vi "Target.vi"   [LabVIEW 2025]
uses:
  <vilib>/eio/utilities/niEioResolveVilibRelativePath.vi
  <vilib>/rvi/interface/RandomDataEmulation/niFpgaRandomDataHandleErrors.vi
  <vilib>/rvi/Memory/Memory_Emulation/nirvimemoryFastEmulation.vi
  <vilib>/rvi/Memory/Memory_Emulation/nirvimemoryEmulation.vi
  <vilib>/rvi/Emulation/niFpgaEmulationIsFPGAContextNoSignature.vi
  <vilib>/rvi/DataTransferAndStorage/Container/Common/niFpgaContainerGetUniqueNameForEmu.vi
  <vilib>/rvi/Emulation/niFpgaProcessEmulError.vi
  <vilib>/rvi/Emulation/niFpgaSctlEmulationGetInTimedLoop.vi
  <vilib>/rvi/errors/nirviReportUnexpectedCaseInternalError (U32).vi
  <vilib>/ARTS-Lab/Array-based Linear Algebra/vector_matrix_multiply_VIs/vector_matrix_multiply_SGL.vi
  <vilib>/ARTS-Lab/Array-based Linear Algebra/matrix_matrix_VIs/matrix_matrix_multiply_SGL.vi
  <vilib>/rvi/DataTransferAndStorage/Container/XNode/niFpgaContainer.xnode
  <vilib>/rvi/interface/RandomDataEmulation/nirviRandomDataFpgaReadWriteTemplate.vi
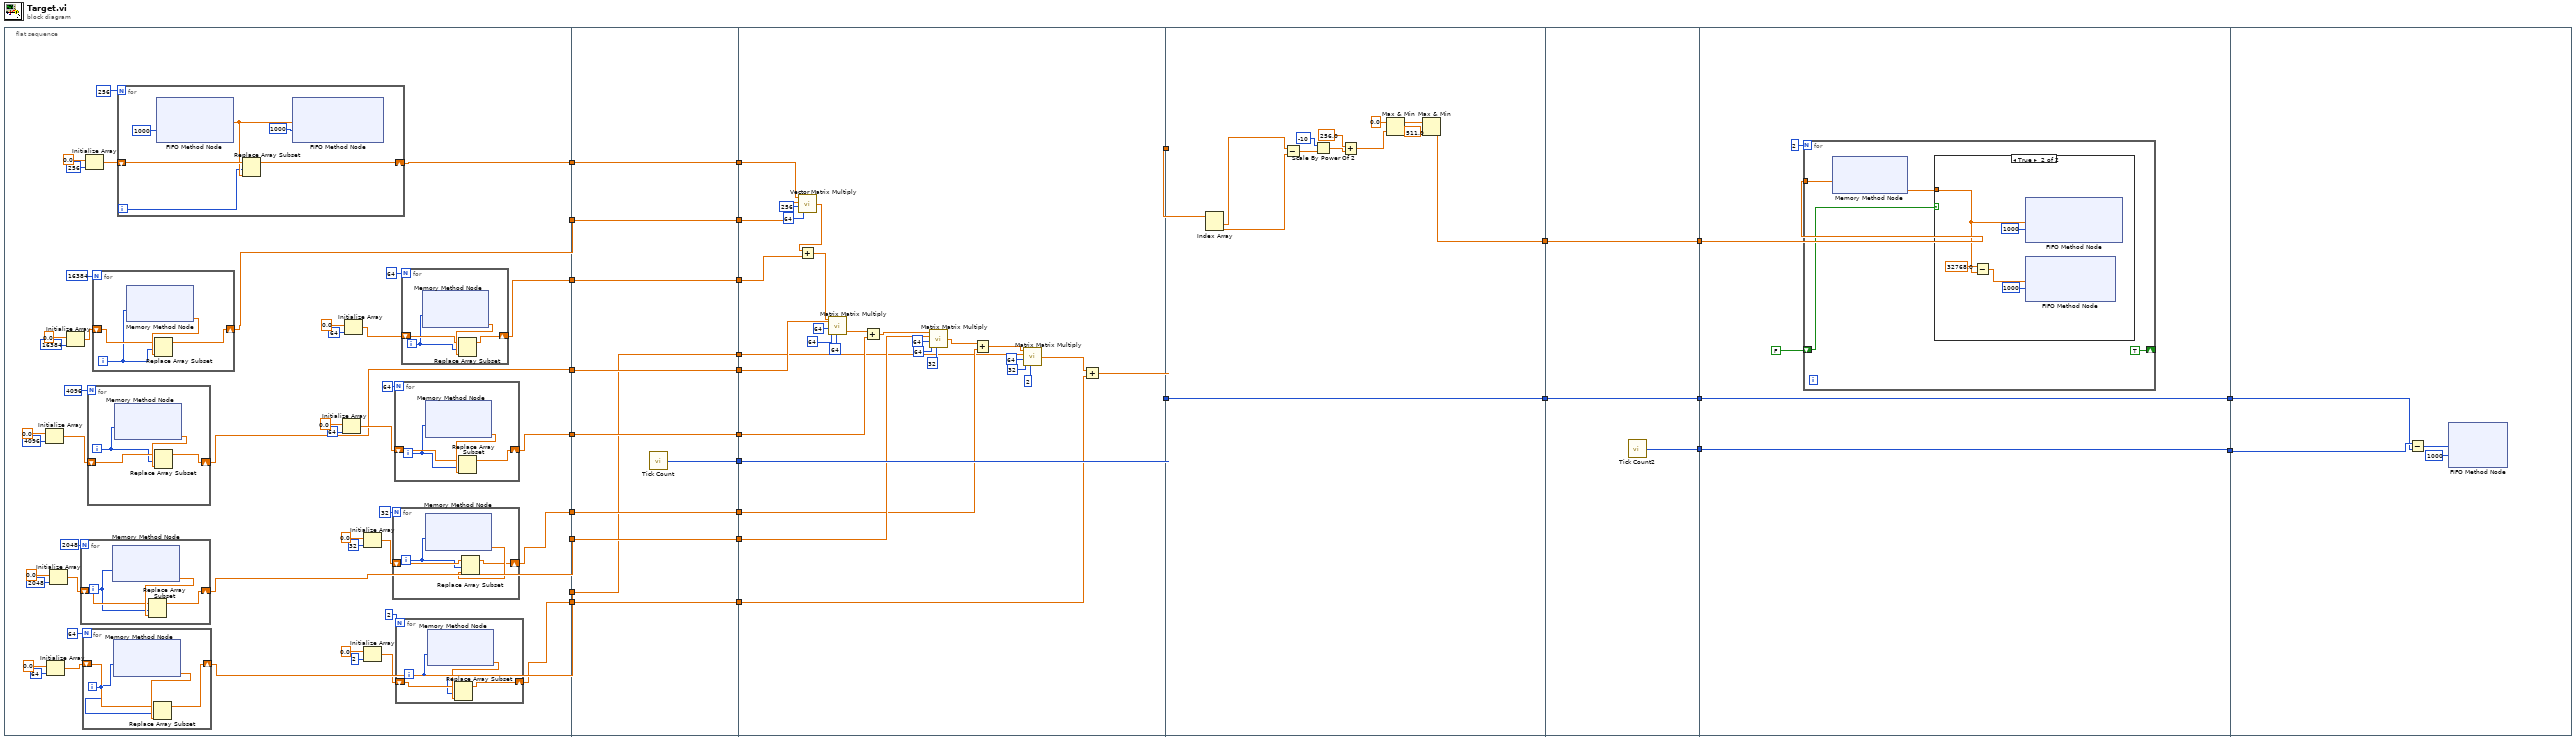
[diagram p0: block diagram]
diagram:
  n1 = flat-sequence {
    tunnel: [w72] -> w19
    tunnel: [w58] -> w17
    tunnel: [w41] -> w15
    tunnel: [w36] -> w13
    tunnel: [w40] -> w11
    tunnel: [w39] -> w8
    tunnel: [w33] -> w6
    tunnel: [w35] -> w4
    tunnel: [w34] -> w1
    tunnel: w19 -> [w121]
    tunnel: [w121] -> w18
    tunnel: w17 -> [w120]
    tunnel: [w120] -> w16
    tunnel: w15 -> [w119]
    tunnel: [w119] -> w14
    tunnel: w13 -> [w118]
    tunnel: [w118] -> w12
    tunnel: w11 -> [w117]
    tunnel: [w117] -> w10
    tunnel: [w116] -> w9
    tunnel: w8 -> [w115]
    tunnel: [w115] -> w7
    tunnel: w6 -> [w114]
    tunnel: [w114] -> w5
    tunnel: w4 -> [w113]
    tunnel: [w113] -> w3
    tunnel: [w112] -> w2
    tunnel: w1 -> [w112]
    tunnel: [w122] -> w28
    tunnel: [w150] -> w27
    tunnel: w9 -> [w150]
    tunnel: w10 -> [w139]
    tunnel: w12 -> [w147]
    tunnel: w14 -> [w141]
    tunnel: w16 -> [w148]
    tunnel: w18 -> [w149]
    tunnel: w7 -> [w136]
    tunnel: w5 -> [w130]
    tunnel: w3 -> [w126]
    tunnel: w2 -> [w125]
    tunnel: w28 -> [w153]
    tunnel: [w152] -> w26
    tunnel: w27 -> [w151]
    tunnel: [w151] -> w25
    tunnel: w26 -> [w166]
    tunnel: [w166] -> w24
    tunnel: w25 -> [w165]
    tunnel: [w165] -> w23
    tunnel: [w164] -> w22
    tunnel: w24 -> [w170]
    tunnel: [w167] -> w21
    tunnel: w23 -> [w168]
    tunnel: [w168] -> w20
    tunnel: w22 -> [w167]
    tunnel: w21 -> [w184]
    tunnel: w20 -> [w183]
    frame #0 {
      n2 = Initialize Array(sgl 0.0 ("element"), 4096 ("dimension size")) -> (w30:sgl[])
      n3 = Initialize Array(sgl 0.0 ("element"), 64 ("dimension size")) -> (w29:sgl[])
      n4 = Initialize Array(sgl 0.0 ("element"), 2048 ("dimension size")) -> (w38:sgl[])
      n5 = Initialize Array(sgl 0.0 ("element"), 16384 ("dimension size")) -> (w57:sgl[])
      n6 = for {
        N: 2048 -> [_]
        shift-right: [w88] -> w39
        shift-left: w38 -> [w87]
        i -> [w86]
        n7 = xnode ("Memory Method Node")("Address"=w86) -> ("Data"=w89:sgl)  [unwired: 1 in, 1 out]
        n8 = Replace Array Subset(array=w87, new element=w89, index=w86) -> (w88:sgl[])
      }
      n9 = for {
        N: 64 -> [_]
        shift-right: [w80] -> w35
        shift-left: w29 -> [w79]
        i -> [w78]
        n10 = xnode ("Memory Method Node")("Address"=w78) -> ("Data"=w81:sgl)  [unwired: 1 in, 1 out]
        n11 = Replace Array Subset(array=w79, new element=w81, index=w78) -> (w80:sgl[])
      }
      n12 = Initialize Array(sgl 0.0 ("element"), 256 ("dimension size")) -> (w69:sgl[])
      n13 = for {
        N: 4096 -> [_]
        shift-right: [w96] -> w36
        shift-left: w30 -> [w95]
        i -> [w94]
        n14 = xnode ("Memory Method Node")("Address"=w94) -> ("Data"=w97:sgl)  [unwired: 1 in, 1 out]
        n15 = Replace Array Subset(array=w95, new element=w97, index=w94) -> (w96:sgl[])
      }
      n16 = for {
        N: 16384 -> [_]
        shift-right: [w105] -> w58
        shift-left: w57 -> [w103]
        i -> [w102]
        n17 = xnode ("Memory Method Node")("Address"=w102) -> ("Data"=w104:sgl)  [unwired: 1 in, 1 out]
        n18 = Replace Array Subset(array=w103, new element=w104, index=w102) -> (w105:sgl[])
      }
      n19 = for {
        N: 256 -> [_]
        shift-right: [w107] -> w72
        shift-left: w69 -> [w109]
        i -> [w106]
        n20 = xnode ("FIFO Method Node")("Timeout"=1000) -> ("Element"=w108:sgl)  [unwired: 1 in, 2 out]
        n21 = Replace Array Subset(array=w109, new element=w108, index=w106) -> (w107:sgl[])
        n22 = xnode ("FIFO Method Node")("Element"=w108, "Timeout"=1000) -> ()  [unwired: 1 in, 2 out]
      }
      n23 = Initialize Array(sgl 0.0 ("element"), 64 ("dimension size")) -> (w37:sgl[])
      n24 = Initialize Array(sgl 0.0 ("element"), 64 ("dimension size")) -> (w42:sgl[])
      n25 = Initialize Array(sgl 0.0 ("element"), 32 ("dimension size")) -> (w31:sgl[])
      n26 = Initialize Array(sgl 0.0 ("element"), 2 ("dimension size")) -> (w32:sgl[])
      n27 = for {
        N: 32 -> [_]
        shift-right: [w83] -> w33
        shift-left: w31 -> [w84]
        i -> [w82]
        n28 = xnode ("Memory Method Node")("Address"=w82) -> ("Data"=w85:sgl)  [unwired: 1 in, 1 out]
        n29 = Replace Array Subset(array=w84, new element=w85, index=w82) -> (w83:sgl[])
      }
      n30 = for {
        N: 64 -> [_]
        shift-right: [w91] -> w40
        shift-left: w37 -> [w92]
        i -> [w90]
        n31 = xnode ("Memory Method Node")("Address"=w90) -> ("Data"=w93:sgl)  [unwired: 1 in, 1 out]
        n32 = Replace Array Subset(array=w92, new element=w93, index=w90) -> (w91:sgl[])
      }
      n33 = for {
        N: 2 -> [_]
        shift-right: [w75] -> w34
        shift-left: w32 -> [w76]
        i -> [w74]
        n34 = xnode ("Memory Method Node")("Address"=w74) -> ("Data"=w77:sgl)  [unwired: 1 in, 1 out]
        n35 = Replace Array Subset(array=w76, new element=w77, index=w74) -> (w75:sgl[])
      }
      n36 = for {
        N: 64 -> [_]
        shift-right: [w99] -> w41
        shift-left: w42 -> [w100]
        i -> [w98]
        n37 = xnode ("Memory Method Node")("Address"=w98) -> ("Data"=w101:sgl)  [unwired: 1 in, 1 out]
        n38 = Replace Array Subset(array=w100, new element=w101, index=w98) -> (w99:sgl[])
      }
    }
    frame #1 {
      n39 = call "Tick Count"() -> ("Tick Count(uSec)"=w116:u32)
    }
    frame #2 {
      n40 = call-poly <vilib>:"Vector Matrix Multiply.vi"("p"=64, "n"=256, "B"=w148, "A"=w149) -> ("C"=w142:sgl[])
      n41 = Add(x=w142, y=w141) -> (x+y=w140:sgl[])
      n42 = call-poly <vilib>:"Matrix Matrix Multiply.vi"("p"=64 ("n"), "n"=64, "m"=64, "B"=w147, "A"=w140) -> ("C"=w138:sgl[])  [unwired: 1 in]
      n43 = Add(x=w138, y=w139) -> (x+y=w137:sgl[])
      n44 = call-poly <vilib>:"Matrix Matrix Multiply.vi"("p"=32, "n"=64, "m"=64, "B"=w136, "A"=w137) -> ("C"=w131:sgl[])  [unwired: 1 in]
      n45 = Add(x=w131, y=w130) -> (x+y=w127:sgl[])
      n46 = call-poly <vilib>:"Matrix Matrix Multiply.vi"("p"=2, "n"=32, "m"=64, "B"=w126, "A"=w127) -> ("C"=w124:sgl[])  [unwired: 1 in]
      n47 = Add(x=w124, y=w125) -> (x+y=w122:sgl[])
    }
    frame #3 {
      n48 = Index Array(array=w153) -> (element #1=w158:sgl, element #2=w159:sgl)  [unwired: 2 in]
      n49 = Subtract(x=w158, y=w159) -> (x-y=w160:sgl)
      n50 = Scale By Power Of 2(n=i16 -10, x=w160) -> (x*2^n=w161:sgl)
      n51 = Add(x=sgl 256.0, y=w161) -> (x+y=w162:sgl)
      n52 = Max & Min(x=sgl 0.0, y=w162) -> (max(x,y)=w163:sgl)  [unwired: 1 out]
      n53 = Max & Min(x=w163, y=sgl 511.0) -> (min(x,y)=w152:sgl)  [unwired: 1 out]
    }
    frame #4 {
      n54 = call "Tick Count2"() -> ("Tick Count(uSec)"=w164:u32)
    }
    frame #5 {
      n55 = for {
        N: 2 -> [_]
        tunnel: w170 -> [w175]
        shift-right: [TRUE] -> _
        shift-left: FALSE -> [w174]
        n56 = xnode ("Memory Method Node")("Address"=w175) -> ("Data"=w172:sgl)  [unwired: 1 in, 1 out]
        n57 = case shown="True" w174 {
          tunnel: w172 -> [_ w176]
          frame False {
          }
          frame True {
            n58 = Subtract(x=sgl 32768.0, y=w176) -> (x-y=w180:sgl)
            n59 = xnode ("FIFO Method Node")("Element"=w176, "Timeout"=1000) -> ()  [unwired: 1 in, 2 out]
            n60 = xnode ("FIFO Method Node")("Element"=w180, "Timeout"=1000) -> ()  [unwired: 1 in, 2 out]
          }
        }
      }
    }
    frame #6 {
      n61 = Subtract(x=w184, y=w183) -> (x-y=w182:u32)
      n62 = xnode ("FIFO Method Node")("Element"=w182, "Timeout"=1000) -> ()  [unwired: 1 in, 2 out]
    }
  }
